vi "Clear Comparator Bin.vi"   [LabVIEW 2016, in "Agilent E4980.lvlib"]
doc: "Limit table actions."
uses:
  <instrlib>/Agilent E4980/Agilent E4980.lvlib
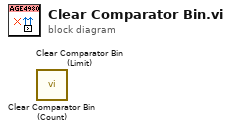
[diagram p0: block diagram]
diagram:
  n1 = call <instrlib>:"Clear Comparator Bin (Count).vi"() -> ()  [unwired: 10 in, 2 out]
  n2 = call <instrlib>:"Clear Comparator Bin (Limit).vi"() -> ()  [unwired: 10 in, 2 out]
